vi "niRFUtil CFG INI File Section.vi"(0 "File In":path, 5 "Section":string, 11 "error in (no error)":errorcluster, 13 "Action (Read)":enum16{"Read", "Write", "Delete"}(ring)) -> (4 "dup File":path, 6 "Key Names":string[](array[string]), 15 "error out":errorcluster)   [LabVIEW 2015, in "niRFUtil.lvlib"]
doc: "The Modify INI File VI allows the user to read or write entries in a text file that is in the standard Windows INI file format. \n\nThe Read action will return an array of strings of all of the Key names in a specified section of the INI file.\n\nThe Write action will create an empty section in the INI file.\n\nThe Delete action will delete the specified section.\n\n(c) Copyright 2007, National Instruments, Inc. This software may not be duplicated, sold, or distributed without written consent from National Instruments."
uses:
  niRFUtil.lvlib
  kernel32.dll
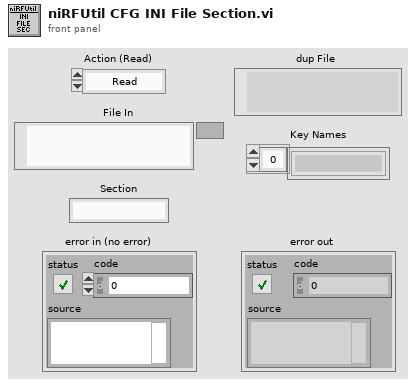
[diagram p1: front panel]
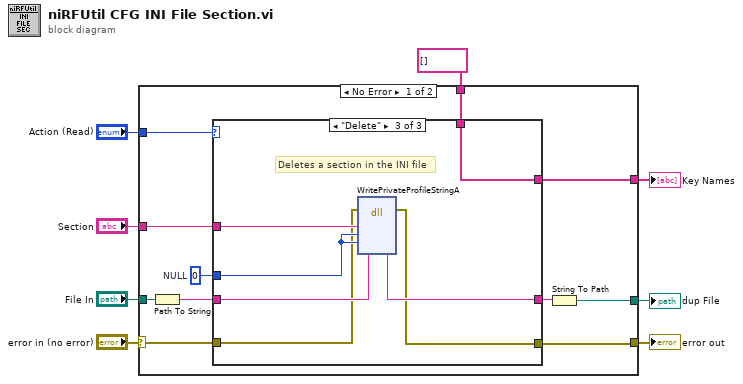
[diagram p0: block diagram]
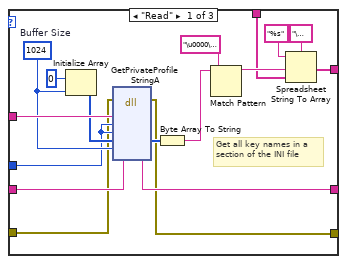
[diagram p2: hidden frame]
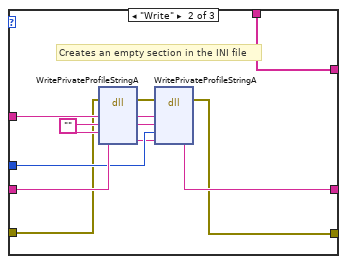
[diagram p3: hidden frame]
diagram:
  n1 = case shown="No Error" "error in (no error)" {
    selector: "error in (no error)" -> [w10 w56]
    tunnel: [w9 w56] -> w8
    tunnel: [w14 w58] -> w3
    tunnel: "Action (Read)" -> [w19 _]
    tunnel: "Section" -> [w18 _]
    tunnel: "File In" -> [w17 w57]
    tunnel: string[] [] ("Key Names") -> [w13 w58]
    tunnel: [w11 w57] -> w2
    frame No Error {
      w12 = 0  # NULL
      n2 = Path To String(path=w17) -> (string=w16:string)
      n3 = case shown="\"Delete\"" w19 {
        tunnel: w18 -> [w36 w48 w55]
        tunnel: w16 -> [w29 w47 w54]
        tunnel: [w28 w40 w53] -> w15
        tunnel: [w24 w46 w52] -> w14
        tunnel: w13 -> [w23 w46 w52]
        tunnel: w12 -> [w22 w44 w51]
        tunnel: w10 -> [w21 w39 w50]
        tunnel: [w20 w37 w49] -> w9
        frame "Read" {
          w31 = 1024  # Buffer Size
          # "Get all key names in a section of the INI file"
          n4 = Initialize Array(u8 0, w31) -> (w30:u8[])
          n5 = dll-call lib="Kernel32.dll" fn="GetPrivateProfileStringA" label="Read"(error in=w21, "AppName"=w36, "KeyName"=w22, "Default"=w22, "ReturnedString"=w30, "Size"=w31, "FileName"=w29) -> (error out=w20:errorcluster, "ReturnedString"=w35:u8[], "FileName"=w28:string)  [unwired: 6 in, 2 out]
          n6 = Byte Array To String(unsigned byte array=w35) -> (string=w34:string)
          n7 = Match Pattern(string=w34, regular expression="\u0000\u0000") -> (before substring=w27:string)  [unwired: 4 out]
          n8 = Spreadsheet String To Array(delimiter (Tab)="\u0000", format string="%s", spreadsheet string=w27, array type (2D Dbl)=w23) -> (array=w24:string[])
        }
        frame "Write" {
          w45 = ""
          # "Creates an empty section in the INI file"
          n9 = dll-call lib="Kernel32.dll" fn="WritePrivateProfileStringA" label="Write"(error in=w39, "AppName"=w48, "KeyName"=w45, "String"=w45, "FileName"=w47) -> (error out=w38:errorcluster, "AppName"=w42:string, "KeyName"=w43:string, "FileName"=w41:string)  [unwired: 2 in, 3 out]
          n10 = dll-call lib="Kernel32.dll" fn="WritePrivateProfileStringA" label="Write"(error in=w38, "AppName"=w42, "KeyName"=w43, "String"=w44, "FileName"=w41) -> (error out=w37:errorcluster, "FileName"=w40:string)  [unwired: 5 in, 2 out]
        }
        frame "Delete" {
          # "Deletes a section in the INI file"
          n11 = dll-call lib="Kernel32.dll" fn="WritePrivateProfileStringA" label="Delete"(error in=w50, "AppName"=w55, "KeyName"=w51, "String"=w51, "FileName"=w54) -> (error out=w49:errorcluster, "FileName"=w53:string)  [unwired: 5 in, 2 out]
        }
      }
      n12 = String To Path(string=w15) -> (path=w11:path)
    }
    frame Error {
    }
  }
  "error out" <- w8
  "Key Names" <- w3
  "dup File" <- w2
